vi "Text to UTF-8 -placeContent.vi"   [LabVIEW 2017]
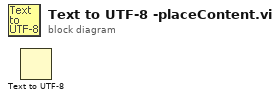
[diagram p0: block diagram]
diagram:
  n1 = Text to UTF-8() -> ()  [unwired: 3 in, 2 out]
